vi "ADB-Serial_WrRd.vi"(4 "flow control (0:none)":u16(ring) items=["None", "XON/XOFF", "RTS/CTS", "XON/XOFF & RTS/CTS", "DTR/DSR", "XON/XOFF & DTR/DSR"], 5 "ReadInterval(mSec)":u32=75, 6 "Tx Deay":u16 max=250 step=5, 7 "Timeout(Sec)":dbl=5.0, 8 "error in (no error)":errorcluster, 9 "PassString":string="***", 10 "Command":string="***", 11 "ComPort":refnum<visa-resource-name>="COM10") -> (0 "error out":errorcluster, 2 "PASS":bool, 3 "received":string)   [LabVIEW 2018]
uses:
  <vilib>/Instr/_visa.llb/VISA Configure Serial Port (Instr).vi
panel:
  out "concatenated string":string
  # "ADB Serial W/R"
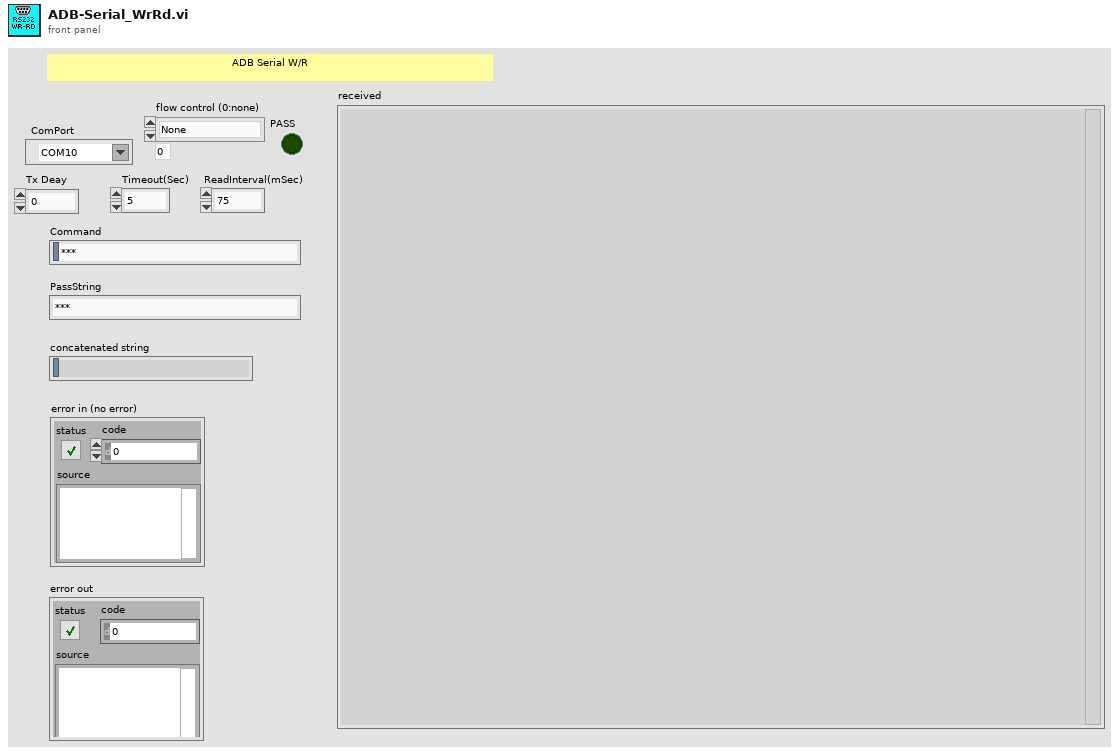
[diagram p1: front panel]
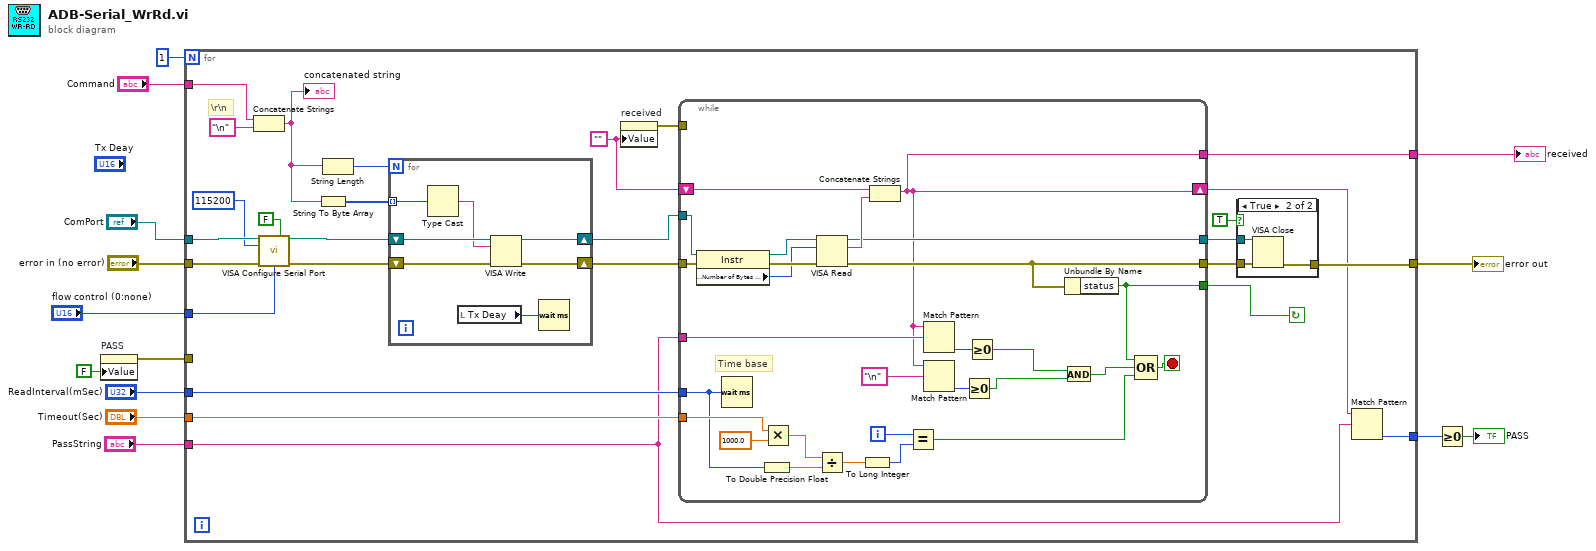
[diagram p0: block diagram]
diagram:
  n1 = property on="PASS" class="Bool (strict)"("Value"=FALSE ("PASS")) -> (error out=w4:errorcluster)  [unwired: 2 in, 1 out]
  n2 = for {
    N: 1 -> [_]
    tunnel: "ComPort" -> [w41]
    tunnel: "ReadInterval(mSec)" -> [w40]
    tunnel: [w39] -> w11
    tunnel: "Timeout(Sec)" -> [w34]
    tunnel: "PassString" -> [w29]
    tunnel: "Command" -> [w25]
    tunnel: "error in (no error)" -> [w38]
    tunnel: [w33] -> w5
    tunnel: w4 -> [_]
    tunnel: [w16] -> w2
    tunnel: "flow control (0:none)" -> [w15]
    stop <- w22 continue-if-true
    w20 = ""
    # "\\r\\n"
    n3 = Concatenate Strings(w25, "\n" ("string")) -> (w18:string)
    "concatenated string" <- w18
    n4 = call-poly "VISA Configure Serial Port"("VISA resource name"=w41, "Enable Termination\nChar (T)"=FALSE ("Enable Termination\nChar (T)"), "baud rate (9600)"=u32 115200 ("Serial Settings:Baud Rate"), "error in (no error)"=w38, "flow control (0:none)"=w15) -> ("VISA resource name out"=w36:refnum<visa-resource-name>, "error out"=w35:errorcluster)  [unwired: 9 in]
    n5 = String To Byte Array(string=w18) -> (unsigned byte array=w19:u8[])
    n6 = String Length(string=w18) -> (length=w17:i32)
    n7 = for {
      N: w17 -> [_]
      shift-right: [w46] -> w30
      shift-left: w36 -> [w48]
      shift-right: [w45] -> w23
      shift-left: w35 -> [w47]
      tunnel: w19 -> [w44] mode=indexing
      n8 = Type Cast(x=w44) -> (*(type *) &x=w43:string)  [unwired: 1 in]
      n9 = local read "Tx Deay"() -> (w42:u16)
      n10 = VISA Write(VISA resource name=w48, write buffer=w43, error in (no error)=w47) -> (VISA resource name out=w46:refnum<visa-resource-name>, error out=w45:errorcluster)  [unwired: 1 out]
      n11 = Wait (ms)(milliseconds to wait=w42) -> ()  [unwired: 1 out]
    }
    n12 = property on="received" class="Str"("Value"=w20) -> (error out=w24:errorcluster)  [unwired: 2 in, 1 out]
    n13 = while {
      tunnel: w23 -> [w80]
      tunnel: w30 -> [w79]
      tunnel: [w55] -> w31
      shift-right: [w53] -> w26
      shift-left: w20 -> [w76]
      tunnel: [w74] -> w32
      tunnel: w40 -> [w67]
      tunnel: w34 -> [w70]
      tunnel: w29 -> [w61]
      tunnel: [w54] -> w22
      tunnel: w24 -> [_]
      tunnel: [w53] -> w16
      i -> [w71]
      stop <- w73 stop-if-true
      # "Time base"
      n14 = property class="Instr"(reference=w79, error in=w80) -> (reference out=w77:refnum<visa-resource-name>, error out=w78:errorcluster, "Serial Settings:Number of Bytes at Serial Port"=w63:u32)
      n15 = Wait (ms)(milliseconds to wait=w67) -> ()  [unwired: 1 out]
      n16 = To Double Precision Float(number=w67) -> (double precision float=w64:dbl)
      n17 = Multiply(x=w70, y=1000.0) -> (x*y=w68:dbl)
      n18 = VISA Read(VISA resource name=w77, byte count=w63, error in (no error)=w78) -> (VISA resource name out=w74:refnum<visa-resource-name>, read buffer=w75:string, error out=w55:errorcluster)  [unwired: 1 out]
      n19 = Divide(x=w68, y=w64) -> (x/y=w66:dbl)
      n20 = To Long Integer(number=w66) -> (32bit integer=w65:i32)
      n21 = Concatenate Strings(w76, w75) -> (w53:string)
      n22 = Equal?(x=w71, y=w65) -> (x = y?=w72:bool)
      n23 = Match Pattern(string=w53, regular expression=w61) -> (offset past match=w62:i32)  [unwired: 1 in, 3 out]
      n24 = Match Pattern(string=w53, regular expression="\n") -> (offset past match=w60:i32)  [unwired: 1 in, 3 out]
      n25 = Greater Or Equal To 0?(x=w60) -> (x >= 0?=w56:bool)
      n26 = Greater Or Equal To 0?(x=w62) -> (x >= 0?=w57:bool)
      n27 = And(x=w57, y=w56) -> (x .and. y?=w59:bool)
      n28 = Unbundle By Name(w55) -> ("status"=w54:bool)
      n29 = Compound Arithmetic op=OR(w54, w59, w72) -> (w73:bool)
    }
    n30 = case shown="True" TRUE {
      tunnel: [w49 w52] -> w33
      tunnel: w32 -> [_ w51]
      tunnel: w31 -> [w49 w50]
      frame False {
      }
      frame True {
        n31 = VISA Close(VISA resource name=w51, error in (no error)=w50) -> (error out=w52:errorcluster)
      }
    }
    n32 = Match Pattern(string=w26, regular expression=w29) -> (offset past match=w39:i32)  [unwired: 1 in, 3 out]
  }
  "error out" <- w5
  "received" <- w2
  n33 = Greater Or Equal To 0?(x=w11) -> (x >= 0?=→"PASS":bool)
